vi "Configure Harmonics.vi"(0 "VISA resource name":refnum<visa-resource-name>, 1 "PLL Source (0: U1)":i32(ring) items=["U1", "I1", "U2", "I2", "U3", "I3", "U4", "I4", "U5", "I5", "U6", "I6", "External Clock"], 2 "Group (1: Harmonics 1)":i32(ring)=1 items=["Harmonics 1"=1, "Harmonics 2"=2], 5 "Minimum Order (0)":i32 min=0 max=1, 7 "Maximum Order (100)":i32=100 min=1 max=500, 9 "Distortion Factor (0: 1/Total)":i32(ring) items=["1/Total", "1/Fundamental"], 11 "error in (no error)":errorcluster) -> (4 "VISA resource name out":refnum<visa-resource-name>, 15 "error out":errorcluster)   [LabVIEW 2021, in "Yokogawa WT1800 Series.lvlib"]
doc: "Configures the harmonics features.\n\n<b>Note:</b>\nThis setting valid on models with the simultaneous dual harmonic measurement (/G6) option or the harmonic measurement (/G5) option."
uses:
  <instrlib>/Yokogawa WT1800 Series/Yokogawa WT1800 Series.lvlib
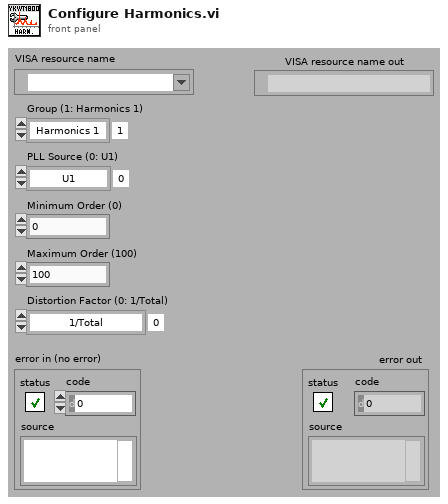
[diagram p1: front panel]
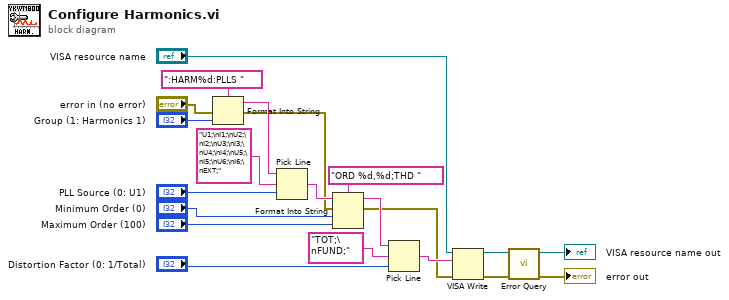
[diagram p0: block diagram]
diagram:
  n1 = Format Into String(format string=":HARM%d:PLLS " ("形式文字列"), error in="error in (no error)", "Group (1: Harmonics 1)") -> (resulting string=w10:string, error out=w6:errorcluster)  [unwired: 1 in]
  n2 = Pick Line ("ライン選択")(string ("")=w10, multi-line string="U1;\nI1;\nU2;\nI2;\nU3;\nI3;\nU4;\nI4;\nU5;\nI5;\nU6;\nI6;\nEXT;" ("複数行文字列"), line index="PLL Source (0: U1)") -> (output string=w8:string)
  n3 = Format Into String(format string="ORD %d,%d;THD " ("形式文字列"), initial string=w8, error in=w6, "Minimum Order (0)", "Maximum Order (100)") -> (resulting string=w2:string, error out=w1:errorcluster)
  n4 = Pick Line ("ライン選択")(string ("")=w2, multi-line string="TOT;\nFUND;" ("複数行文字列"), line index="Distortion Factor (0: 1/Total)") -> (output string=w15:string)
  n5 = VISA Write ("VISA書き込み")(VISA resource name="VISA resource name", write buffer=w15, error in (no error)=w1) -> (VISA resource name out=w21:refnum<visa-resource-name>, error out=w20:errorcluster)  [unwired: 1 out]
  n6 = call <instrlib>:"Error Query.vi"("error in (no error)"=w20, "VISA resource name"=w21) -> ("error out"=→"error out":errorcluster, "VISA resource name out"=→"VISA resource name out":refnum<visa-resource-name>)  [unwired: 6 in, 2 out]
